vi "REV Functions.vi"() -> ()   [LabVIEW 2026]
uses:
  vi.lib/Custom Controls/c_Spark_APIVersion.ctl
  vi.lib/REVLibDriver5/REVLibDriver.lvlib
panel:
  out "c_Spark_APIVersion":T1
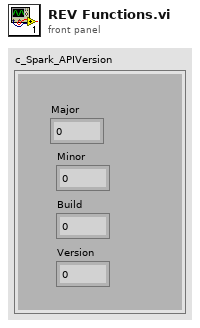
[diagram p1: front panel]
types:
  T1 = typedef "REVLibDriver.lvlib/c_Spark_APIVersion.ctl" = cluster{"Major":u16, "Minor":u8, "Build":u8, "Version":u32}
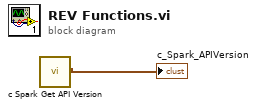
[diagram p0: block diagram]
diagram:
  n1 = call "c Spark Get API Version.vi"() -> ("c_Spark_APIVersion"=→"c_Spark_APIVersion":T1)  [unwired: 9 in, 2 out]
